vi "FPGA_CounterConvertEdgeTypeToMode.vi"(11 "EdgeType":T3={"Master Mode"=enum."Edge Detection", "UpChannel"=enum."Disabled", "DownChannel"=enum."Disabled", "High/Up"=FALSE}) -> (2 "Mode":T1, 3 "Edges":T2)   [LabVIEW 2017]
uses:
  <vilib>/Rock Robotics/SystemInterfaces/Counter/FPGA_CounterCtrEdgeDetectionType.ctl
  <vilib>/Rock Robotics/SystemInterfaces/Counter/FPGA_CounterEventCtrMode.ctl
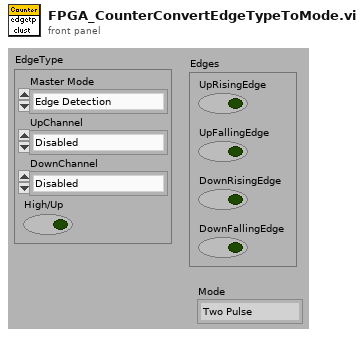
[diagram p1: front panel]
types:
  T1 = typedef "FPGA_CounterEventCtrMode.ctl" = enum8{"Two Pulse", "Semiperiod", "Pulse Length", "External Direction"}
  T2 = cluster{"UpRisingEdge":bool, "UpFallingEdge":bool, "DownRisingEdge":bool, "DownFallingEdge":bool}
  T3 = typedef "FPGA_CounterCtrEdgeDetectionType.ctl" = cluster{"Master Mode":enum16{"Edge Detection", "Semi Period Mode", "Pulse Length Mode", "External Direction"}, "UpChannel":enum16{"Rising Edge", "Falling Edge", "Raising & Falling Edge", "Disabled"}, "DownChannel":enum16{"Rising Edge", "Falling Edge", "Raising & Falling Edge", "Disabled"}, "High/Up":bool}
  T4 = enum16{"Edge Detection", "Semi Period Mode", "Pulse Length Mode", "External Direction"}
  T5 = enum16{"Rising Edge", "Falling Edge", "Raising & Falling Edge", "Disabled"}
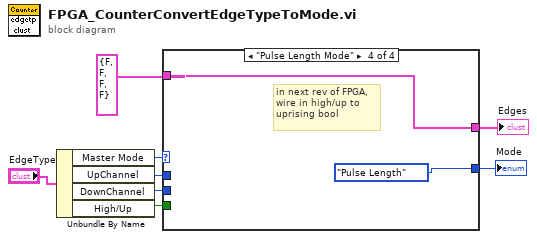
[diagram p0: block diagram]
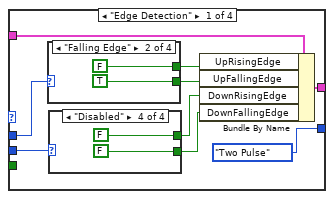
[diagram p2: hidden frame]
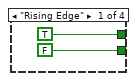
[diagram p3: hidden frame]
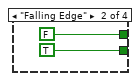
[diagram p4: hidden frame]
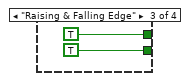
[diagram p5: hidden frame]
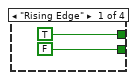
[diagram p6: hidden frame]
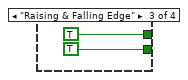
[diagram p7: hidden frame]
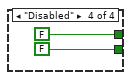
[diagram p8: hidden frame]
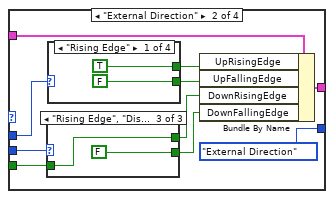
[diagram p9: hidden frame]
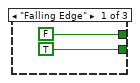
[diagram p10: hidden frame]
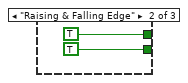
[diagram p11: hidden frame]
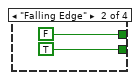
[diagram p12: hidden frame]
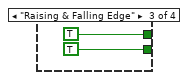
[diagram p13: hidden frame]
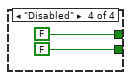
[diagram p14: hidden frame]
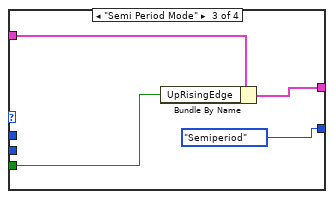
[diagram p15: hidden frame]
diagram:
  n1 = Unbundle By Name("EdgeType") -> ("Master Mode"=w7:T4, "UpChannel"=w6:T5, "DownChannel"=w5:T5, "High/Up"=w1:bool)
  n2 = case shown="\"Pulse Length Mode\"" w7 {
    tunnel: T2 {"UpRisingEdge"=FALSE, "UpFallingEdge"=FALSE, "DownRisingEdge"=FALSE, "DownFallingEdge"=FALSE} ("Edges") -> [w17 w43 w61 w62]
    tunnel: [w16 w42 w60 w62] -> w3
    tunnel: w6 -> [w15 w41 _ _]
    tunnel: w5 -> [w12 w37 _ _]
    tunnel: [FPGA_CounterEventCtrMode."Two Pulse" ("Mode") FPGA_CounterEventCtrMode."External Direction" ("Mode") FPGA_CounterEventCtrMode."Semiperiod" ("Mode") FPGA_CounterEventCtrMode."Pulse Length" ("Mode")] -> w4
    tunnel: w1 -> [_ w36 w58 _]
    frame "Edge Detection" {
      n3 = case shown="\"Falling Edge\"" w15 {
        tunnel: [TRUE FALSE TRUE FALSE] -> w14
        tunnel: [FALSE TRUE TRUE FALSE] -> w13
        frame "Rising Edge" {
        }
        frame "Falling Edge" {
        }
        frame "Raising & Falling Edge" {
        }
        frame "Disabled" {
        }
      }
      n4 = case shown="\"Disabled\"" w12 {
        tunnel: [TRUE FALSE TRUE FALSE] -> w11
        tunnel: [FALSE TRUE TRUE FALSE] -> w10
        frame "Rising Edge" {
        }
        frame "Falling Edge" {
        }
        frame "Raising & Falling Edge" {
        }
        frame "Disabled" {
        }
      }
      n5 = Bundle By Name(cluster=w17, "UpRisingEdge"=w14, "UpFallingEdge"=w13, "DownRisingEdge"=w11, "DownFallingEdge"=w10) -> (w16:T2)
    }
    frame "External Direction" {
      n6 = case shown="\"Rising Edge\", \"Disabled\"" w37 {
        tunnel: [FALSE TRUE w48] -> w35
        tunnel: [TRUE TRUE FALSE] -> w34
        tunnel: w36 -> [_ _ w48]
        frame "Falling Edge" {
        }
        frame "Raising & Falling Edge" {
        }
        frame "Rising Edge", "Disabled" {
        }
      }
      n7 = case shown="\"Rising Edge\"" w41 {
        tunnel: [TRUE FALSE TRUE FALSE] -> w40
        tunnel: [FALSE TRUE TRUE FALSE] -> w39
        frame "Rising Edge" {
        }
        frame "Falling Edge" {
        }
        frame "Raising & Falling Edge" {
        }
        frame "Disabled" {
        }
      }
      n8 = Bundle By Name(cluster=w43, "UpRisingEdge"=w40, "UpFallingEdge"=w39, "DownRisingEdge"=w35, "DownFallingEdge"=w34) -> (w42:T2)
    }
    frame "Semi Period Mode" {
      n9 = Bundle By Name(cluster=w61, "UpRisingEdge"=w58) -> (w60:T2)
    }
    frame "Pulse Length Mode" {
      # "in next rev of FPGA,\nwire in high/up to \nuprising bool"
    }
  }
  "Edges" <- w3
  "Mode" <- w4
